vi "Enumerate Item Contents.vi"(11 "ProjectItem Refnum":refnum<vi>) -> (3 "Nested Items":T1[](array[typedef]))   [LabVIEW 2018, in "LVClassByRef.lvlib"]
uses:
  <resource>/Framework/Providers/LVClassByRef/LVClassByRef.lvlib
  <resource>/Framework/Providers/LVClassByRef/Enumerated Item.ctl
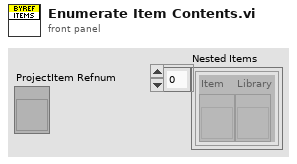
[diagram p1: front panel]
types:
  T1 = typedef "LVClassByRef.lvlib/Enumerated Item.ctl" = cluster{"Item":refnum<vi>, "Library":refnum<vi>}
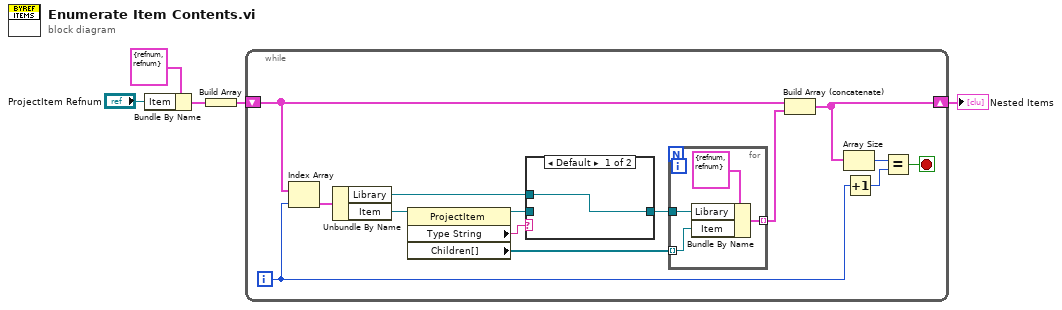
[diagram p0: block diagram]
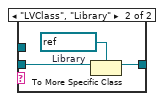
[diagram p2: hidden frame]
diagram:
  n1 = Bundle By Name(cluster=T1 {"Item"=refnum, "Library"=refnum} ("Enumerated Item"), "Item"="ProjectItem Refnum") -> (w3:T1)
  n2 = Build Array(w3) -> (w2:T1[])
  n3 = while {
    shift-right: [w6] -> w1
    shift-left: w2 -> [w8]
    i -> [w16]
    stop <- w17 stop-if-true
    n4 = Index Array(array=w8, index=w16) -> (element=w15:T1)
    n5 = Unbundle By Name(w15) -> ("Library"=w11:refnum<vi>, "Item"=w14:refnum<vi>)
    n6 = property class="ProjectItem"(reference=w14) -> (reference out=w12:refnum<vi>, "Type String"=w13:string, "Children[]"=w9:refnum<vi>[])  [unwired: 1 in, 1 out]
    n7 = case shown="Default" w13 {
      tunnel: w12 -> [_ w27]
      tunnel: w11 -> [w24 _]
      tunnel: [w24 w25] -> w10
      frame Default {
      }
      frame "LVClass", "Library" {
        w26 = refnum<vi> refnum  # Library
        n8 = To More Specific Class(target class=w26, reference=w27) -> (specific class reference=w25:refnum<vi>)  [unwired: 1 in, 1 out]
      }
    }
    n9 = for {
      tunnel: w10 -> [w22]
      tunnel: w9 -> [w21] mode=indexing
      tunnel: [w20] -> w7 mode=indexing
      n10 = Bundle By Name(cluster=T1 {"Item"=refnum, "Library"=refnum} ("Enumerated Item"), "Library"=w22, "Item"=w21) -> (w20:T1)
    }
    n11 = Build Array (concatenate)(w8, w7) -> (w6:T1[])
    n12 = Array Size(array=w6) -> (size(s)=w19:i32)
    n13 = Increment(x=w16) -> (x+1=w18:i32)
    n14 = Equal?(x=w19, y=w18) -> (x = y?=w17:bool)
  }
  "Nested Items" <- w1
